vi "Untitled 3.vi"() -> ()   [LabVIEW 2019]
panel:
  out "concatenated string":string
  out "time string":string
  out "date string":string
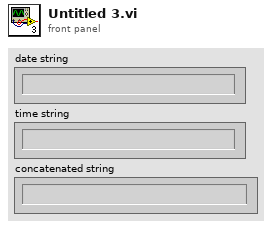
[diagram p1: front panel]
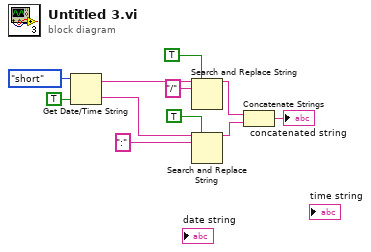
[diagram p0: block diagram]
diagram:
  n1 = Get Date/Time String(date format (0)=enum16{"short", "long", "abbreviated"}."short", want seconds? (F)=TRUE) -> (date string=w5:string, time string=w4:string)  [unwired: 1 in]
  n2 = Search and Replace String(replace all?=TRUE ("replace all? (F)"), input string=w5, search string="/") -> (result string=w3:string)  [unwired: 5 in, 3 out]
  n3 = Search and Replace String(replace all?=TRUE ("replace all? (F)"), input string=w4, search string=":") -> (result string=w2:string)  [unwired: 5 in, 3 out]
  n4 = Concatenate Strings(w3, w2) -> (→"concatenated string":string)
